vi "Close Files.vi"(8 "error in (no error)":errorcluster, 10 "State":T11, 11 "Frame Grabber Data in":T1) -> (0 "error out":errorcluster, 1 "Shutdown?":bool, 2 "File Path Control":path, 3 "Frame Grabber Data Out":T1={"Camera Session"="", "Frame"=refnum, "AVI Refnum"=refnum, "Codecs"=[], "Frame number"=0, "Tracking File Refnum"=refnum, "Tick Count"=0, "Probe Object"=refnum, "Playback Probe Data"=[], "Rigid Body"={"Position"={"x (mm)"=0.0, "y (mm)"=0.0, "z (mm)"=0.0}, "Orientation"={"Pitch (rad)"=0.0, "Yaw (rad)"=0.0, "Roll (rad)"=0.0}, "Quaternion"={"qx"=0.0, "qy"=0.0, "qz"=0.0, "qw"=0.0}, "Tracked?"=FALSE}, "Total no frames playback"=0, "Video FPS"=0.0, "Camera connected?"=FALSE, "Scene"=refnum, "Cropped Frame"=refnum, "Tracker FPS"=0.0, "Crop ROI"=[], "Presentation Values"=[], "Elapsed time (ms)"=0, "Camera frames playback"=0, "Refnums"={"Live Refnum"=refnum, "Record Refnum"=refnum, "Playback Refnum"=refnum, "Frame Slider Refnum"=refnum, "Pause Refnum"=refnum, "Home Refnum"=refnum, "Set Crop Refnum"=refnum, "Clear Crop Refnum"=refnum, "stop refnum"=refnum, "Playback Rate Refnum"=refnum, "Presentation Refnum"=refnum, "Crop Time Frame Slider Refnum"=refnum, "Cancel Save Refnum"=refnum, "Reverse Playback Refnum"=refnum, "Recording Settings Refnum"=refnum, "Continuous Playback Refnum"=refnum, "Annotation Refnum"=refnum, "Export All Refnum"=refnum, "Export List Refnum"=refnum, "Fill List Refnum"=refnum, "Save Crop Refnum"=refnum, "Skip Forward Refnum"=refnum, "Skip Backward Refnum"=refnum, "Single Annotation Refnum"=refnum, "Load Refnum"=refnum, "Set Start Refnum"=refnum, "Set End Refnum"=refnum, "Add to List Refnum"=refnum, "List of Annotations Refnum"=refnum, "Camera Frame Refnum"=refnum}, "Dimensions"={"Probe Dimensions"={"Probe Width"=0.0, "Probe Depth"=1.0, "Probe Height"=0.0}, "Room Dimensions"={"Room Width"=0.0, "Room Depth"=0.0, "Room Height"=0.0}}, "Playback Data As Strings"=[], "Cropped Tracking File Refnum"=refnum, "Cropped AVI Refnum"=refnum, "Header"=[], "Total euclidian distance"=0.0, "Annotation File Path"=path "", "Playback File Path"=path "", "Size per frame"=0.0, "Ground Truth File Refnum"=refnum, "Annotation Array"=[], "Annotation TIFFs Folder"=path "", "overwriting open file?"=FALSE})   [LabVIEW 2017]
uses:
  Controls/Crop Video State.ctl
  Controls/Frame Grabber Data.ctl
  <vilib>/userdefined/High Color/IMAQdx.ctl
  <vilib>/vision/Image Controls.llb/IMAQ Image.ctl
  <vilib>/vision/Avi.llb/IMAQ AVI2 Refnum.ctl
  Controls/Rigid Body Info.ctl
  Controls/Position.ctl
  Controls/Orientation.ctl
  Controls/Refnums.ctl
  Controls/Recording Settings.ctl
  Controls/Operator Settings.ctl
  Controls/Operator.ctl
  Controls/Patient Settings.ctl
  Controls/Dimensions.ctl
  Controls/Room Dimensions.ctl
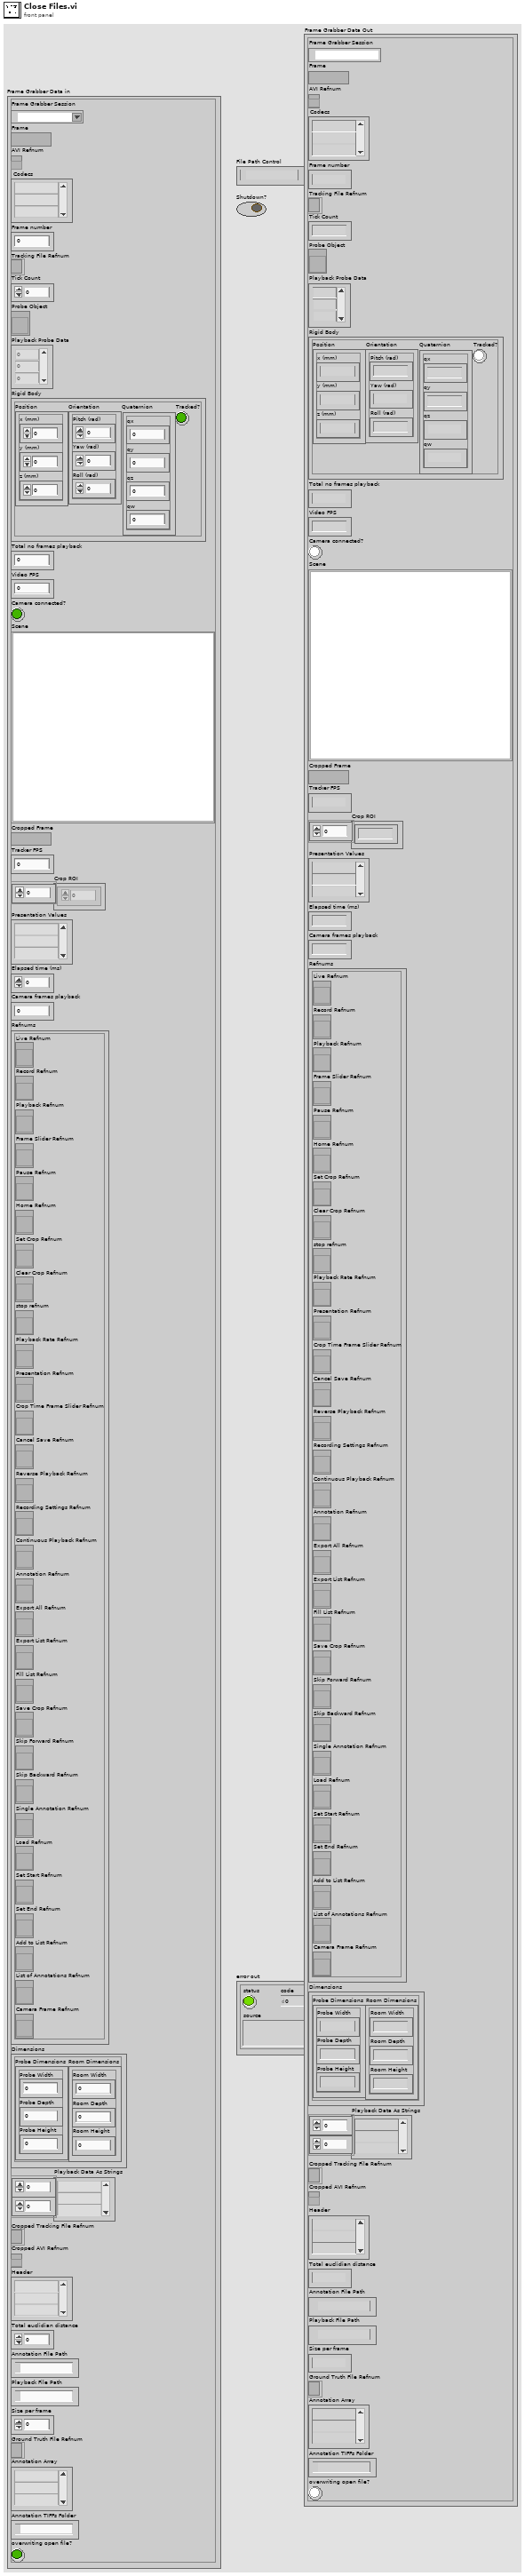
[diagram p1: front panel]
types:
  T1 = typedef "Frame Grabber Data.ctl" = cluster{"Camera Session":T2, "Frame":T3, "AVI Refnum":T4, "Codecs":string[], "Frame number":u32, "Tracking File Refnum":refnum<file>, "Tick Count":u32, "Probe Object":refnum<vi>, "Playback Probe Data":dbl[][], "Rigid Body":T5, "Total no frames playback":i32, "Video FPS":dbl, "Camera connected?":bool, "Scene":refnum<vi>, "Cropped Frame":T3, "Tracker FPS":dbl, "Crop ROI":i32[], "Presentation Values":string[], "Elapsed time (ms)":u32, "Camera frames playback":u32, "Refnums":T8, "Dimensions":T9, "Playback Data As Strings":string[][], "Cropped Tracking File Refnum":refnum<file>, "Cropped AVI Refnum":T4, "Header":string[], "Total euclidian distance":dbl, "Annotation File Path":path, "Playback File Path":path, "Size per frame":dbl, "Ground Truth File Refnum":refnum<file>, "Annotation Array":string[], "Annotation TIFFs Folder":path, "overwriting open file?":bool}
  T2 = typedef "IMAQdx.ctl" = refnum<k21>
  T3 = typedef "IMAQ Image.ctl" = refnum<image>
  T4 = typedef "IMAQ AVI2 Refnum.ctl" = refnum<k20>
  T5 = typedef "Rigid Body Info.ctl" = cluster{"Position":T6, "Orientation":T7, "Quaternion":cluster{"qx":sgl, "qy":sgl, "qz":sgl, "qw":sgl}, "Tracked?":bool}
  T6 = typedef "Position.ctl" = cluster{"x (mm)":sgl, "y (mm)":sgl, "z (mm)":sgl}
  T7 = typedef "Orientation.ctl" = cluster{"Pitch (rad)":sgl, "Yaw (rad)":sgl, "Roll (rad)":sgl}
  T8 = typedef "Refnums.ctl" = cluster{"Live Refnum":refnum<vi>, "Record Refnum":refnum<vi>, "Playback Refnum":refnum<vi>, "Frame Slider Refnum":refnum<vi>, "Pause Refnum":refnum<vi>, "Home Refnum":refnum<vi>, "Set Crop Refnum":refnum<vi>, "Clear Crop Refnum":refnum<vi>, "stop refnum":refnum<vi>, "Playback Rate Refnum":refnum<vi>, "Presentation Refnum":refnum<vi>, "Crop Time Frame Slider Refnum":refnum<vi>, "Cancel Save Refnum":refnum<vi>, "Reverse Playback Refnum":refnum<vi>, "Recording Settings Refnum":refnum<vi>, "Continuous Playback Refnum":refnum<vi>, "Annotation Refnum":refnum<vi>, "Export All Refnum":refnum<vi>, "Export List Refnum":refnum<vi>, "Fill List Refnum":refnum<vi>, "Save Crop Refnum":refnum<vi>, "Skip Forward Refnum":refnum<vi>, "Skip Backward Refnum":refnum<vi>, "Single Annotation Refnum":refnum<vi>, "Load Refnum":refnum<vi>, "Set Start Refnum":refnum<vi>, "Set End Refnum":refnum<vi>, "Add to List Refnum":refnum<vi>, "List of Annotations Refnum":refnum<vi>, "Camera Frame Refnum":refnum<vi>}
  T9 = typedef "Dimensions.ctl" = cluster{"Probe Dimensions":cluster{"Probe Width":sgl, "Probe Depth":sgl, "Probe Height":sgl}, "Room Dimensions":T10}
  T10 = typedef "Room Dimensions.ctl" = cluster{"Room Width":dbl, "Room Depth":dbl, "Room Height":dbl}
  T11 = typedef "Crop Video State.ctl" = enum16{"Init", "Wait", "Load", "Playback Frame", "Save", "Export List", "Export All", "Close", "Set Crop Area", "Reset Crop Area", "Crop Inside", "Crop Outside", "Multi-Crop", "Re-Open Files", "Annotate Frame", "Annotate Clip", "Add to List", "Fill List", "Set Start", "Set End", "Error Handling", "Shutdown"}
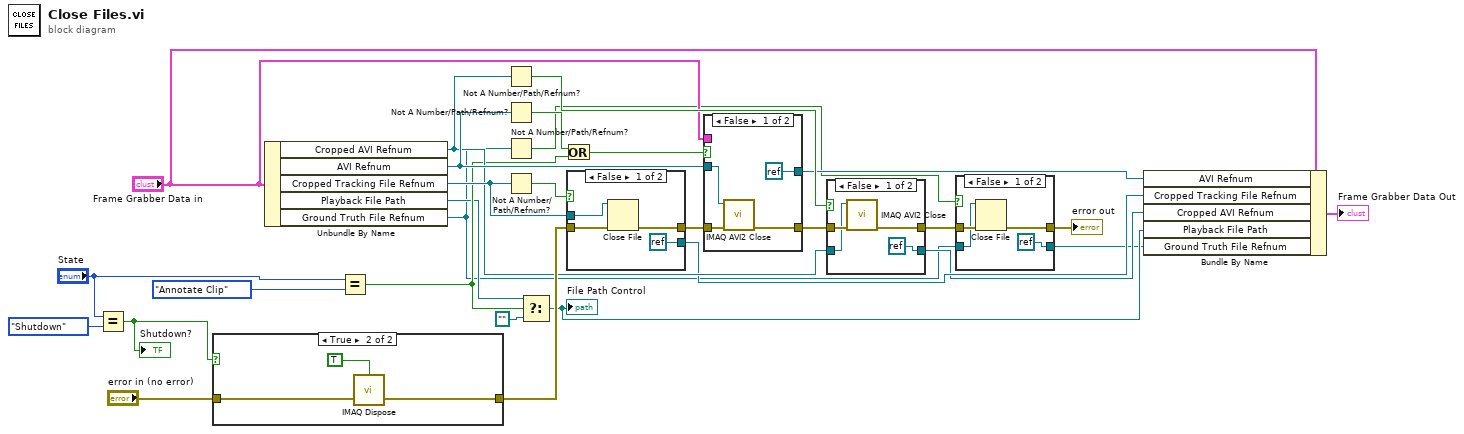
[diagram p0: block diagram]
diagram:
  n1 = Equal?(x="State", y=Crop_Video_State."Shutdown") -> (x = y?=w14:bool)
  "Shutdown?" <- w14
  n2 = case shown="True" w14 {
    tunnel: "error in (no error)" -> [w30 w33]
    tunnel: [w30 w32] -> w28
    frame False {
    }
    frame True {
      n3 = call "IMAQ Dispose"("All Images? (No)"=TRUE, "error in (no error)"=w33) -> ("error out"=w32:errorcluster)  [unwired: 4 in]
    }
  }
  n4 = Unbundle By Name("Frame Grabber Data in") -> ("Cropped AVI Refnum"=w20:T4, "AVI Refnum"=w25:T4, "Cropped Tracking File Refnum"=w23:refnum<file>, "Playback File Path"=w8:path, "Ground Truth File Refnum"=w1:refnum<file>)
  n5 = Equal?(x="State", y=Crop_Video_State."Annotate Clip") -> (x = y?=w9:bool)
  n6 = Not A Number/Path/Refnum?(number/path/refnum=w20) -> (NaN/Path/Refnum?=w19:bool)
  n7 = Not A Number/Path/Refnum?(number/path/refnum=w25) -> (NaN/Path/Refnum?=w26:bool)
  n8 = Not A Number/Path/Refnum?(number/path/refnum=w1) -> (NaN/Path/Refnum?=w5:bool)
  n9 = Not A Number/Path/Refnum?(number/path/refnum=w23) -> (NaN/Path/Refnum?=w22:bool)
  n10 = Select(t=w8, s=w9, f=path "") -> (s? t:f=w6:path)
  "File Path Control" <- w6
  n11 = Or(x=w26, y=w9) -> (x .or. y?=w13:bool)
  n12 = case shown="False" w22 {
    tunnel: w28 -> [w37 w39]
    tunnel: [w36 w39] -> w24
    tunnel: w23 -> [w35 w38]
    tunnel: [refnum<k0> refnum w38] -> w17
    frame False {
      n13 = Close File(refnum=w35, error in=w37) -> (error out=w36:errorcluster)  [unwired: 1 out]
    }
    frame True {
    }
  }
  n14 = case shown="False" w13 {
    tunnel: w24 -> [w43 w45]
    tunnel: [w42 w45] -> w21
    tunnel: w25 -> [w41 w44]
    tunnel: [refnum<k0> refnum w44] -> w15
    tunnel: "Frame Grabber Data in" -> [_ _]
    frame False {
      n15 = call "IMAQ AVI2 Close"("error in (no error)"=w43, "AVI Refnum"=w41) -> ("error out"=w42:errorcluster)  [unwired: 9 in]
    }
    frame True {
    }
  }
  n16 = case shown="False" w19 {
    tunnel: w21 -> [w49 w51]
    tunnel: [w48 w51] -> w4
    tunnel: w20 -> [w47 w50]
    tunnel: [refnum<k0> refnum w50] -> w16
    frame False {
      n17 = call "IMAQ AVI2 Close"("error in (no error)"=w49, "AVI Refnum"=w47) -> ("error out"=w48:errorcluster)  [unwired: 9 in]
    }
    frame True {
    }
  }
  n18 = case shown="False" w5 {
    tunnel: w4 -> [w55 w57]
    tunnel: [w54 w57] -> w3
    tunnel: w1 -> [w53 w56]
    tunnel: [refnum<k0> refnum w56] -> w2
    frame False {
      n19 = Close File(refnum=w53, error in=w55) -> (error out=w54:errorcluster)  [unwired: 1 out]
    }
    frame True {
    }
  }
  "error out" <- w3
  n20 = Bundle By Name(cluster="Frame Grabber Data in", "AVI Refnum"=w15, "Cropped Tracking File Refnum"=w17, "Cropped AVI Refnum"=w16, "Playback File Path"=w6, "Ground Truth File Refnum"=w2) -> (→"Frame Grabber Data Out":T1)
